vi "Initialize.vi"(8 "error in (no error)":errorcluster, 11 "Initial Count (0)":u32) -> (0 "error out":errorcluster, 3 "Count Request Message out":refnum<class "Count Request Message.lvclass">)   [LabVIEW 2017, in "Count Request Message.lvclass"]
uses:
  Count Request Message.lvclass
  Count Request Message.lvclass/Count Request Message.ctl
panel:
  in  "Count Request Message in":refnum<class "Count Request Message.lvclass">
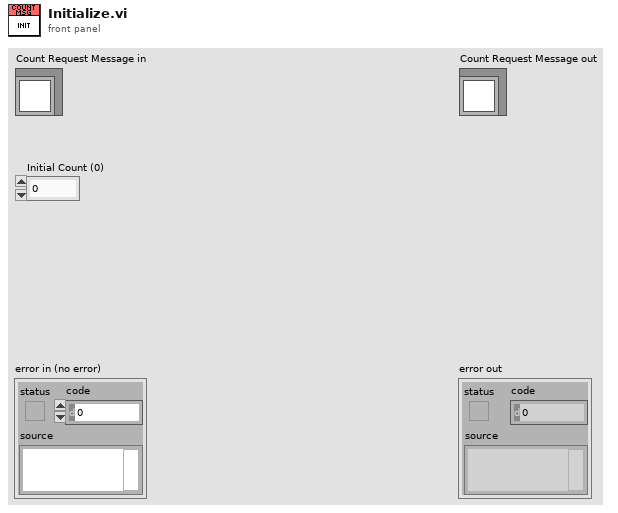
[diagram p1: front panel]
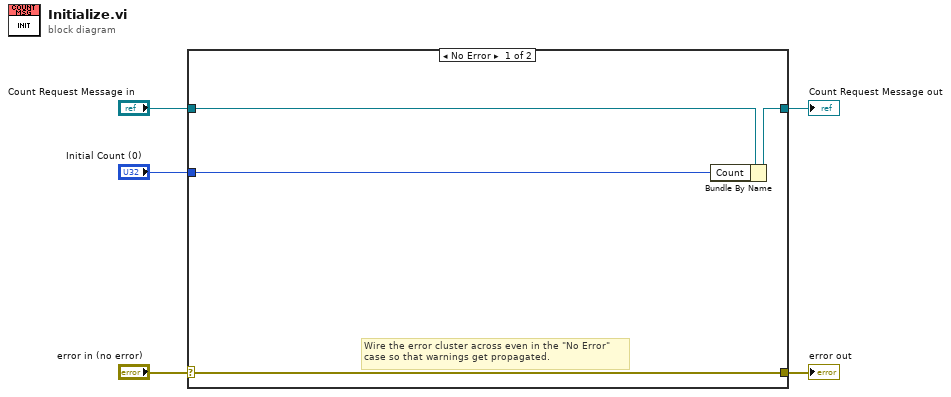
[diagram p0: block diagram]
diagram:
  n1 = case shown="No Error" "error in (no error)" {
    selector: "error in (no error)" -> [w9 w11]
    tunnel: [w9 w11] -> w4
    tunnel: [w6 w10] -> w2
    tunnel: "Count Request Message in" -> [w8 w10]
    tunnel: "Initial Count (0)" -> [w7 _]
    frame No Error {
      # "Wire the error cluster across even in the \"No Error\"\ncase so that warnings get propagated."
      n2 = Bundle By Name(cluster=w8, "Count"=w7) -> (w6:refnum<class "Count Request Message.lvclass">)
    }
    frame Error {
    }
  }
  "error out" <- w4
  "Count Request Message out" <- w2
